vi "Format Rate-Field.vi"(4 "unit":string, 5 "rate":dbl, 6 "unit":string, 7 "field":dbl) -> (1 "ratedisp":string, 3 "fielddisp":string)   [LabVIEW 2009, in "Magnet.lvclass"]
uses:
  Magnet.lvclass
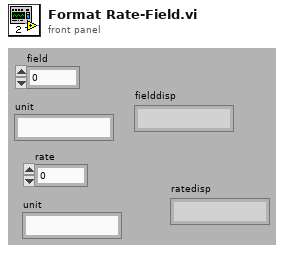
[diagram p1: front panel]
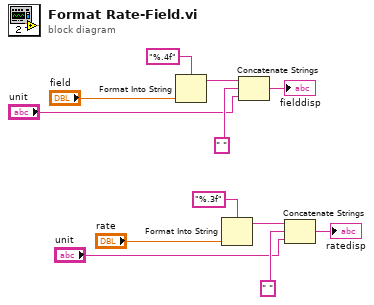
[diagram p0: block diagram]
diagram:
  n1 = Format Into String(format string="%.4f", "field") -> (resulting string=w11:string)  [unwired: 2 in, 1 out]
  n2 = Format Into String(format string="%.3f", "rate") -> (resulting string=w5:string)  [unwired: 2 in, 1 out]
  n3 = Concatenate Strings(w11, " ", "unit") -> (→"fielddisp":string)
  n4 = Concatenate Strings(w5, " ", "unit") -> (→"ratedisp":string)
